vi "Configure Serial Bus (SENT - Fast Signal).vi"(0 "VISA resource name":refnum<visa-resource-name>, 1 "Nibble Order\n(0: Most Significant Nibble First)":u16(ring) items=["Most Significant Nibble First", "Least Significant Nibble First"], 2 "Multiplier (1.0)":dbl=1.0, 3 "Offset (1)":dbl=1.0, 5 "Serial Bus Name (1: Serial Bus 1)":u16(ring)=1 items=["Serial Bus 1"=1, "Serial Bus 2"=2], 7 "Fast Signal (1: Signal 1)":i32(ring)=1 items=["Signal 1"=1, "Signal 2"=2, "Signal 3"=3, "Signal 4"=4, "Signal 5"=5, "Signal 6"=6], 9 "Enable Signal (True)":bool=TRUE, 11 "error in (no error)":errorcluster, 12 "Start Bit (1)":i32=1, 13 "Length (1)":i32=1) -> (4 "VISA resource name out":refnum<visa-resource-name>, 15 "error out":errorcluster)   [LabVIEW 2016, in "Agilent 2000 3000 X-Series.lvlib"]
doc: "Configures setting for fast SENT singnals."
uses:
  Agilent 2000 3000 X-Series.lvlib
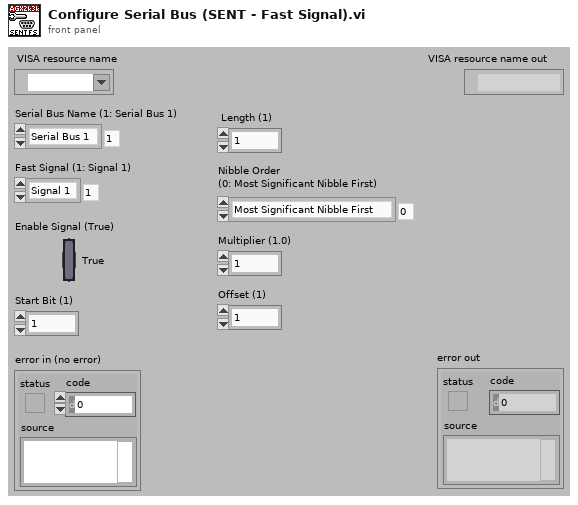
[diagram p1: front panel]
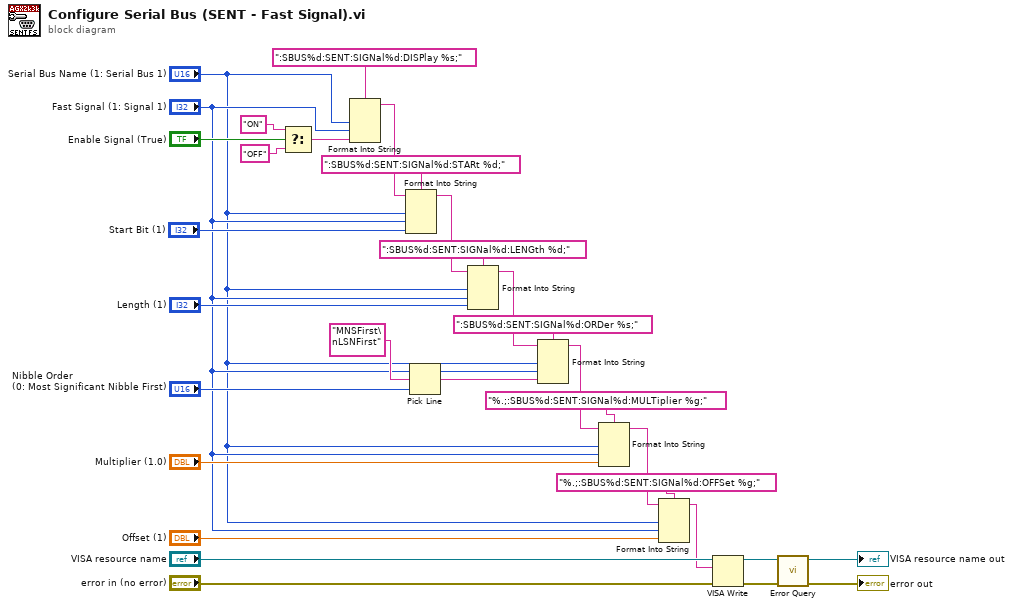
[diagram p0: block diagram]
diagram:
  n1 = Select(t="ON", s="Enable Signal (True)", f="OFF") -> (s? t:f=w27:string)
  n2 = Format Into String(format string=":SBUS%d:SENT:SIGNal%d:DISPlay %s;", "Serial Bus Name (1: Serial Bus 1)", "Fast Signal (1: Signal 1)", w27) -> (resulting string=w24:string)  [unwired: 2 in, 1 out]
  n3 = Format Into String(format string=":SBUS%d:SENT:SIGNal%d:STARt %d;", initial string=w24, "Serial Bus Name (1: Serial Bus 1)", "Fast Signal (1: Signal 1)", "Start Bit (1)") -> (resulting string=w21:string)  [unwired: 1 in, 1 out]
  n4 = Pick Line(multi-line string="MNSFirst\nLSNFirst", line index="Nibble Order\n(0: Most Significant Nibble First)") -> (output string=w18:string)  [unwired: 1 in]
  n5 = Format Into String(format string=":SBUS%d:SENT:SIGNal%d:LENGth %d;", initial string=w21, "Serial Bus Name (1: Serial Bus 1)", "Fast Signal (1: Signal 1)", "Length (1)") -> (resulting string=w19:string)  [unwired: 1 in, 1 out]
  n6 = Format Into String(format string=":SBUS%d:SENT:SIGNal%d:ORDer %s;", initial string=w19, "Serial Bus Name (1: Serial Bus 1)", "Fast Signal (1: Signal 1)", w18) -> (resulting string=w13:string)  [unwired: 1 in, 1 out]
  n7 = Format Into String(format string="%.;:SBUS%d:SENT:SIGNal%d:MULTiplier %g;", initial string=w13, "Serial Bus Name (1: Serial Bus 1)", "Fast Signal (1: Signal 1)", "Multiplier (1.0)") -> (resulting string=w11:string)  [unwired: 1 in, 1 out]
  n8 = Format Into String(format string="%.;:SBUS%d:SENT:SIGNal%d:OFFSet %g;", initial string=w11, "Serial Bus Name (1: Serial Bus 1)", "Fast Signal (1: Signal 1)", "Offset (1)") -> (resulting string=w5:string)  [unwired: 1 in, 1 out]
  n9 = VISA Write(VISA resource name="VISA resource name", write buffer=w5, error in (no error)="error in (no error)") -> (VISA resource name out=w4:refnum<visa-resource-name>, error out=w3:errorcluster)  [unwired: 1 out]
  n10 = call "Error Query.vi"("error in (no error)"=w3, "VISA resource name"=w4) -> ("error out"=→"error out":errorcluster, "VISA resource name out"=→"VISA resource name out":refnum<visa-resource-name>)  [unwired: 6 in, 2 out]
